vi "Check panel run status.vi"(8 "error in (no error)":errorcluster, 11 "Fiber Auto Collimation panel in":refnum<class "Fiber Auto Collimation panel.lvclass">) -> (0 "error out":errorcluster, 1 "Clone names running":string[](array[string]), 2 "Panel(s) running":bool, 3 "Fiber Auto Collimation panel out":refnum<class "Fiber Auto Collimation panel.lvclass">)   [LabVIEW 2018, in "Fiber Auto Collimation panel.lvclass"]
doc: "This VI checks to see if the Panel (or at least one clone, if it's a Panel supporting clones) is running or not.\n\nIf the check returns True, then the \"Clone names running\" array will be populated with a list of the clone names running at the moment. If the Panel does not support clones but the one panel it does allow is running, it returns an array of length 1 with the value of its sole element being an empty string.\n\nThe top-level Panel class will always return True."
uses:
  Fiber Auto Collimation panel.lvclass
  Fiber Auto Collimation panel.lvclass/Fiber Auto Collimation panel.ctl
  <vilib>/Utility/error.llb/Clear Errors.vi
  <userlib>/nLight Error Handling/Log any errors.vi
  <vilib>/Utility/LVClass/Get LV Class Name.vi
  <userlib>/nLight Error Handling/Merge errors no loss.vi
  References/Fiber Auto Collimation References.lvclass
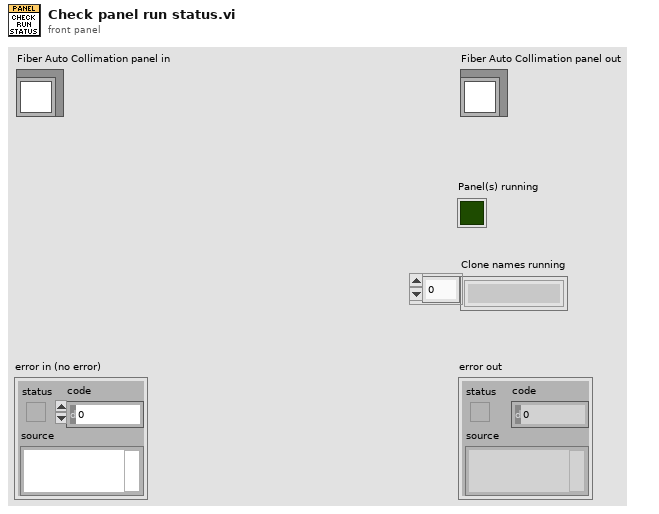
[diagram p1: front panel]
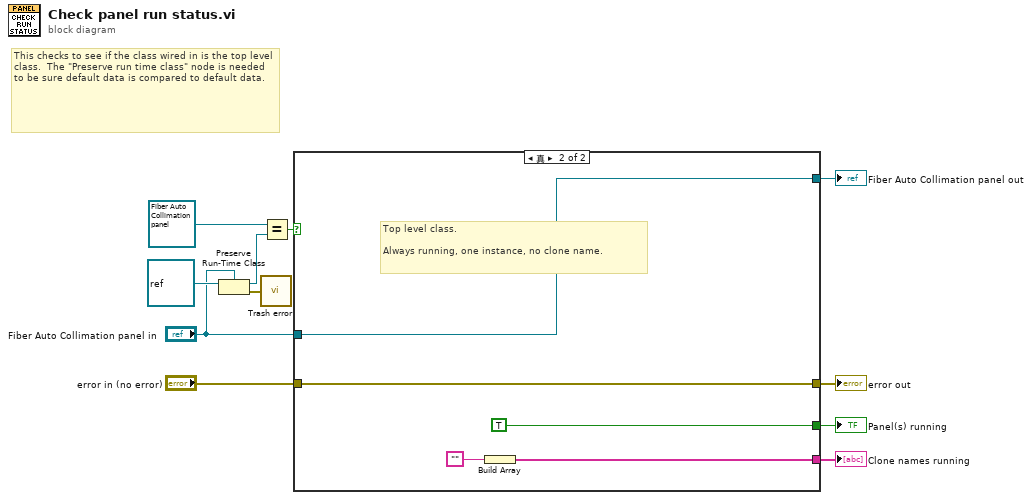
[diagram p0: block diagram]
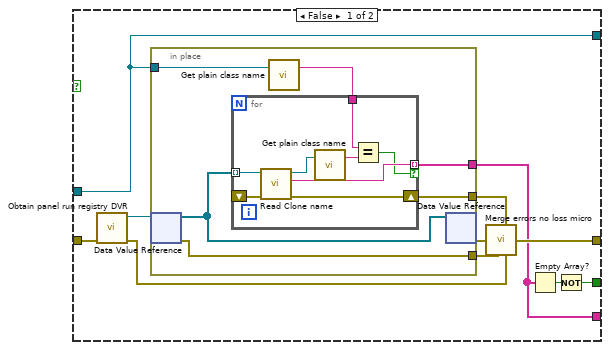
[diagram p2: hidden frame]
diagram:
  # "This checks to see if the class wired in is the top level class.  The \"Preserve run time class\" node is needed to be sure default data is compared to default data."
  n1 = Preserve Run-Time Class(object in=refnum<class> refnum ("LabVIEW Object"), 2:"Fiber Auto Collimation panel in") -> (object out=w7:refnum<class "Fiber Auto Collimation panel.lvclass">, error out=w1:errorcluster)  [unwired: 1 in]
  n2 = call <userlib>:"Trash error.vi"("error in"=w1) -> ()  [unwired: 15 in]
  n3 = Equal?(x=refnum<class "Fiber Auto Collimation panel.lvclass"> refnum ("nLight Station Template panel in"), y=w7) -> (x = y?=w6:bool)
  n4 = case shown="真" w6 {
    tunnel: [w16 w40] -> w11
    tunnel: [w14 TRUE] -> w10
    tunnel: "Fiber Auto Collimation panel in" -> [w12 w38]
    tunnel: [w12 w38] -> w4
    tunnel: "error in (no error)" -> [w13 w37]
    tunnel: [w17 w37] -> w2
    frame False {
      n5 = call "Obtain panel run registry DVR.vi"("error in"=w13) -> ("error out"=w19:errorcluster, "Panel registration DVR"=w22:refnum<data-value>)  [unwired: 9 in]
      n6 = in-place {
        in-place-border: [w28] -> w20
        in-place-border: [w27] -> w18
        in-place-border: w12 -> [w25]
        in-place-border: [w23] -> w16
        n7 = in-place-dvr #1(w22) -> (w24:refnum<class "Fiber Auto Collimation panel.lvclass">[], w28:errorcluster)
        n8 = call <userlib>:"Get plain class name.vi"("Any class"=w25) -> ("Plain class name"=w26:string)  [unwired: 2 in]
        n9 = for {
          tunnel: w24 -> [w36] mode=indexing
          shift-right: [w33] -> w27
          shift-left: _ -> [w34]
          tunnel: w26 -> [w31]
          tunnel: [w30] -> w23 mode=indexing if=w29
          n10 = call "Read Clone name.vi"("error in (no error)"=w34, "Fiber Auto Collimation panel in"=w36) -> ("error out"=w33:errorcluster, "Clone name"=w30:string, "Fiber Auto Collimation panel out"=w35:refnum<class "Fiber Auto Collimation panel.lvclass">)  [unwired: 7 in]
          n11 = call <userlib>:"Get plain class name.vi"("Any class"=w35) -> ("Plain class name"=w32:string)  [unwired: 2 in]
          n12 = Equal?(x=w31, y=w32) -> (x = y?=w29:bool)
        }
        n13 = in-place-dvr #1(w24) -> (w21:errorcluster)  [unwired: 1 out]
      }
      n14 = call <userlib>:"Merge errors no loss micro.vi"("error in (no error) 1"=w21, "error in (no error) 5"=w20, "error in (no error) 3"=w18, "error in (no error) 6"=w19) -> ("error out"=w17:errorcluster)  [unwired: 5 in]
      n15 = Empty Array?(array=w16) -> (empty?=w15:bool)
      n16 = Not(x=w15) -> (.not. x?=w14:bool)
    }
    frame True {
      # "Top level class.\n\nAlways running, one instance, no clone name."
      n17 = Build Array("") -> (w40:string[])
    }
  }
  "error out" <- w2
  "Fiber Auto Collimation panel out" <- w4
  "Clone names running" <- w11
  "Panel(s) running" <- w10
